vi "Set DAC DUC Mode.vi"(0 "fpga interface in":refnum<k20>, 5 "DAC Digital Upconverter Channel":string="AO0", 7 "Enable DAC Digital Upconverter":bool, 11 "error in (no error)":errorcluster) -> (4 "fpga interface out":refnum<k20>, 15 "error out":errorcluster)   [LabVIEW 2018, in "GettingStarted_5785_Host.lvlib"]
uses:
  GettingStarted_5785_Host.lvlib
  <instrlib>/FlexRIO/API/Host/v1/NI FlexRIO/API/Get Property Reference - Fpga Small.vi
  <resource>/objmgr/niflexrioapiChannel.rc
  <instrlib>/FlexRIO/API/Host/v1/NI FlexRIO API v1.lvlib
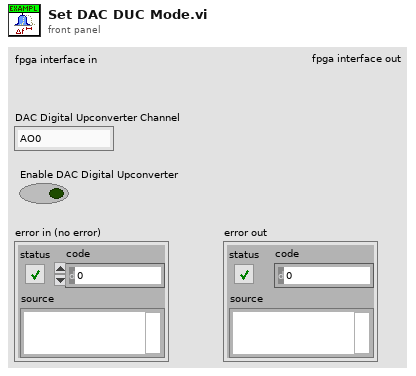
[diagram p1: front panel]
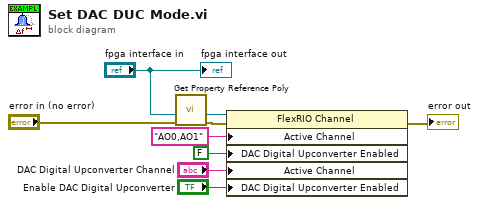
[diagram p0: block diagram]
diagram:
  n1 = call-poly <instrlib>:"Get Property Reference Poly.vi"("error in (no error)"="error in (no error)", "fpga interface in"="fpga interface in") -> ("error out"=w6:errorcluster, "property reference"=w7:refnum<k20>)  [unwired: 4 in, 1 out]
  n2 = property class="FlexRIO Channel"(reference=w7, error in=w6, "Active Channel"="AO0,AO1", "DAC Digital Upconverter Enabled"=FALSE ("Analog Output:DAC Digital Upconverter Enabled"), "Active Channel"="DAC Digital Upconverter Channel", "DAC Digital Upconverter Enabled"="Enable DAC Digital Upconverter") -> (error out=→"error out":errorcluster)  [unwired: 1 out]
  "fpga interface out" <- "fpga interface in"
